vi "STAV Read.vi"(7 "Action (Read)":enum16{"Read", "Init"}(ring), 8 "error in (no error)":errorcluster, 11 "STAV ref in":refnum<visa-resource-name>) -> (0 "error out":errorcluster, 1 "Frame ready":bool, 2 "String":string, 3 "STAV ref out":refnum<visa-resource-name>)   [LabVIEW 2021, in "STAV lib.lvlib"]
uses:
  STAV lib.lvlib
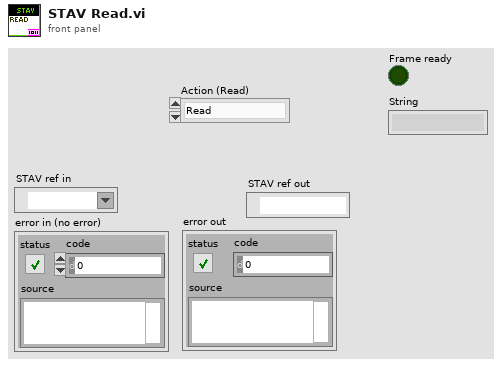
[diagram p1: front panel]
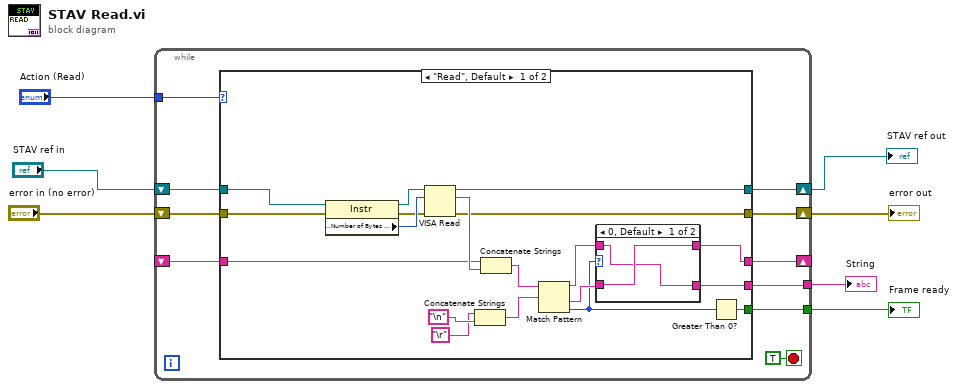
[diagram p0: block diagram]
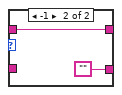
[diagram p2: hidden frame]
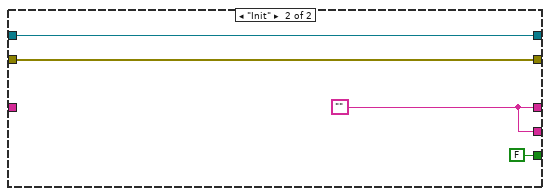
[diagram p3: hidden frame]
diagram:
  n1 = while {
    shift-right: [w15] -> w5
    shift-left: "STAV ref in" -> [w17]
    shift-right: [w14] -> w4
    shift-left: "error in (no error)" -> [w16]
    shift-right: [w12] -> _
    shift-left: _ -> [w13]
    tunnel: "Action (Read)" -> [w10]
    tunnel: [w9] -> w2
    tunnel: [w8] -> w1
    stop <- TRUE stop-if-true
    n2 = case shown="\"Read\", Default" w10 {
      tunnel: w17 -> [w28 w44]
      tunnel: w16 -> [w27 w43]
      tunnel: [w26 w44] -> w15
      tunnel: [w25 w43] -> w14
      tunnel: w13 -> [w24 _]
      tunnel: [w22 w42] -> w12
      tunnel: [w20 w42] -> w9
      tunnel: [w18 FALSE] -> w8
      frame "Read", Default {
        n3 = property class="Instr"(reference=w28, error in=w27) -> (reference out=w36:refnum<visa-resource-name>, error out=w34:errorcluster, "Serial Settings:Number of Bytes at Serial Port"=w35:u32)
        n4 = VISA Read(VISA resource name=w36, byte count=w35, error in (no error)=w34) -> (VISA resource name out=w26:refnum<visa-resource-name>, read buffer=w33:string, error out=w25:errorcluster)  [unwired: 1 out]
        n5 = Concatenate Strings("\r", "\n") -> (w29:string)
        n6 = Concatenate Strings(w24, w33) -> (w32:string)
        n7 = Match Pattern(string=w32, regular expression=w29) -> (before substring=w23:string, after substring=w21:string, offset past match=w19:i32)  [unwired: 1 in, 1 out]
        n8 = case shown="0, Default" w19 {
          tunnel: w23 -> [w37 w40]
          tunnel: [w38 w40] -> w22
          tunnel: w21 -> [w38 _]
          tunnel: [w37 ""] -> w20
          frame 0, Default {
          }
          frame -1 {
          }
        }
        n9 = Greater Than 0?(x=w19) -> (x > 0?=w18:bool)
      }
      frame "Init" {
        w42 = ""
      }
    }
  }
  "STAV ref out" <- w5
  "error out" <- w4
  "String" <- w2
  "Frame ready" <- w1
